vi "Next Message.vi"(7 "Periodic Name (None = Timeout)":string, 8 "error in (no error)":errorcluster, 9 "Timeout/Period ms (-1)":i32=-1, 11 "Module in":refnum<class "Module.lvclass">) -> (0 "error out":errorcluster, 1 "Data":variant, 2 "ID":string, 3 "Module out":refnum<class "Module.lvclass">)   [LabVIEW 2023, in "Volatus.lvlib" / "Module.lvclass"]
uses:
  Module.lvclass
  Module.lvclass/Module.ctl
  MessageQ/MessageQ.lvclass/MessageQ.ctl
  Module Status Update.ctl
  MessageQ/MessageQ.lvclass
  State.ctl
  Module Substatus.ctl
  Metric Update.ctl
  Launch Nested Message.ctl
  VolatusConfig/VolatusConfigElement/VolatusConfigElement.lvclass
  LastAck.ctl
  MessageQ/Send.vi
  Parent Q.vi
  MessageQ/Is Null.vi
  Volatus.lvlib
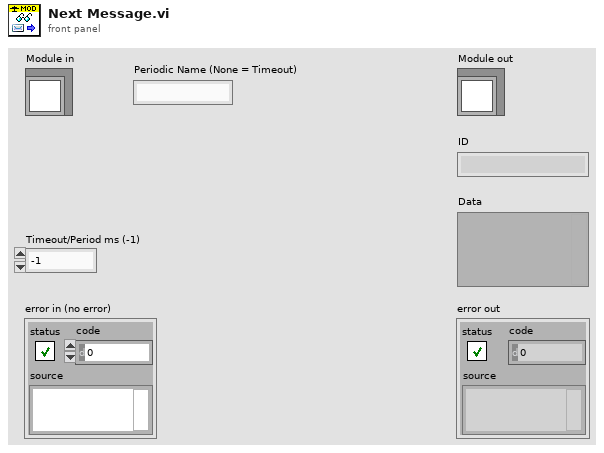
[diagram p1: front panel]
types:
  T1 = typedef "Volatus.lvlib/Metrics Reverse.ctl" = cluster{"End HRS":dbl, "Wait":dbl}
  T2 = typedef "Volatus.lvlib/Metrics Forward.ctl" = cluster{"Name":string, "Start":dbl, "Proc":dbl}
  T3 = typedef "Volatus.lvlib/Module Status Update.ctl" = cluster{"MessageQ":refnum<class "MessageQ.lvclass">, "State":T4, "Hierarchy":string[], "Forwarded":bool}
  T4 = typedef "Volatus.lvlib/Module.lvclass/State.ctl" = enum16{"Unknown", "Launched", "Starting", "Running", "Stopping", "Stopped", "Error - Starting", "Error - Run", "Error - Stopping"}
  T5 = typedef "Volatus.lvlib/Module Substatus.ctl" = cluster{"Hierarchy":string[], "Name":string, "Status":string}
  T6 = typedef "Volatus.lvlib/Metric Update.ctl" = cluster{"Hierarchy":string[], "Name":string, "Value":dbl}
  T7 = typedef "Volatus.lvlib/Launch Nested Message.ctl" = cluster{"Module":refnum<class "Module.lvclass">, "Config":refnum<class "VolatusConfigElement.lvclass">}
  T8 = typedef "Volatus.lvlib/Module.lvclass/LastAck.ctl" = cluster{"Module":refnum<class "Module.lvclass">}
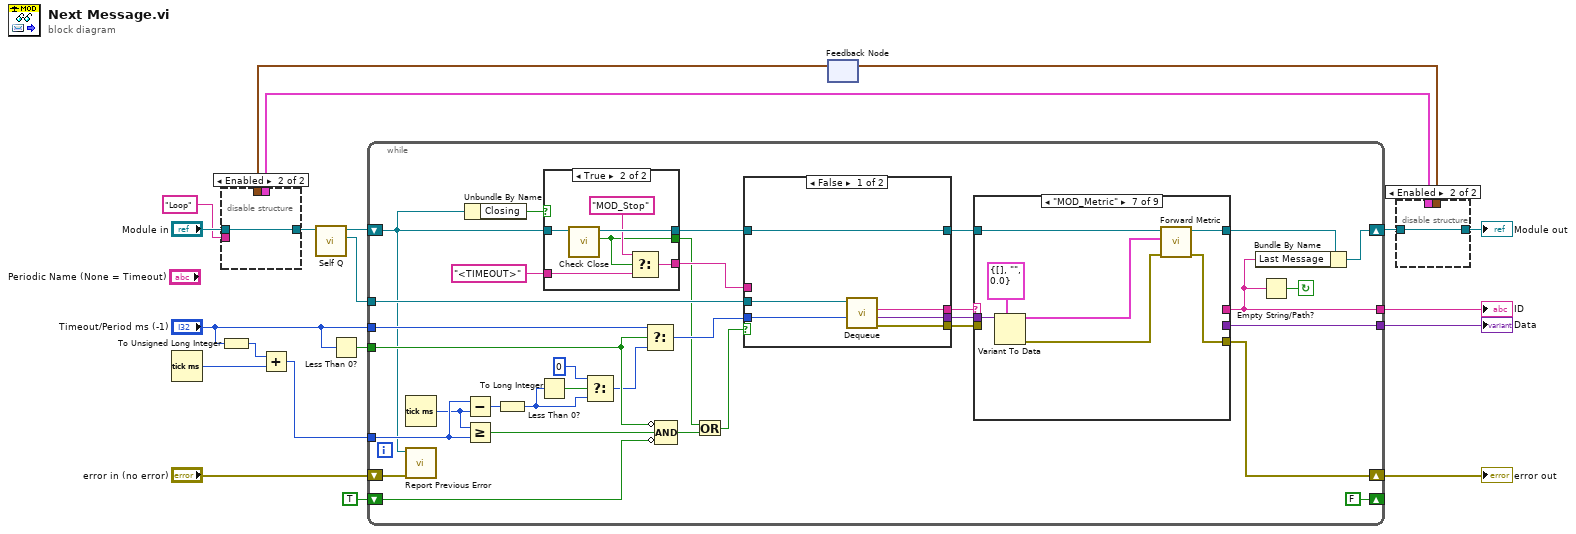
[diagram p0: block diagram]
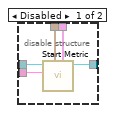
[diagram p2: hidden frame]
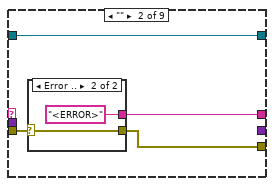
[diagram p6: hidden frame]
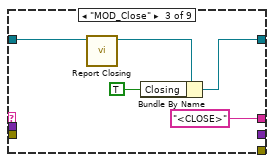
[diagram p8: hidden frame]
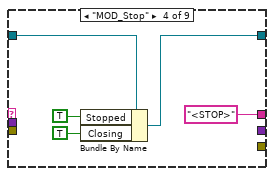
[diagram p9: hidden frame]
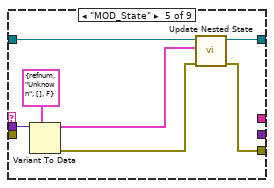
[diagram p10: hidden frame]
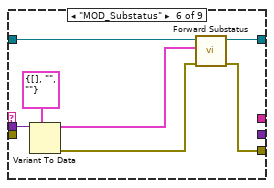
[diagram p11: hidden frame]
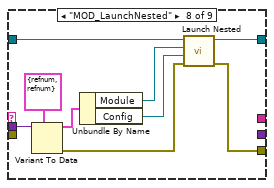
[diagram p12: hidden frame]
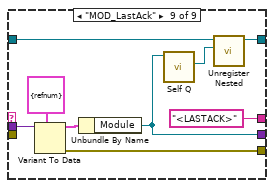
[diagram p13: hidden frame]
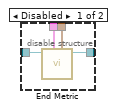
[diagram p14: hidden frame]
diagram:
  n1 = Tick Count (ms)() -> (millisecond timer value=w3:u32)
  n2 = To Unsigned Long Integer(number="Timeout/Period ms (-1)") -> (unsigned 32bit integer=w2:u32)
  n3 = Add(x=w2, y=w3) -> (x+y=w1:u32)
  n4 = Less Than 0?(x="Timeout/Period ms (-1)") -> (x < 0?=w6:bool)
  n5 = feedback #1() -> (w9:T1)  [unwired: 1 in]
  n6 = disable-structure shown="Enabled" {
    disable-tunnel: "Module in" -> [w25 w26]
    disable-tunnel: [w24 w26] -> w14
    disable-tunnel: "Loop" ("Metric") -> [w23 _]
    disable-tunnel: [w22 _] -> w11
    disable-tunnel: w9 -> [w21 _]
    frame Disabled {
      n7 = call "Start Metric.vi"("Metrics Reverse"=w21, "Metric"=w23, "Module in"=w25) -> ("Module out"=w24:refnum<class "Module.lvclass">, "Forward"=w22:T2)  [unwired: 6 in, 1 out]
    }
    frame Enabled {
    }
  }
  n8 = call "Self Q.vi"("Module in"=w14) -> ("Self Q"=w7:refnum<class "MessageQ.lvclass">, "Module out"=w8:refnum<class "Module.lvclass">)  [unwired: 9 in]
  n9 = while {
    shift-right: [w43] -> w15
    shift-left: w8 -> [w32]
    tunnel: w7 -> [w58]
    tunnel: w1 -> [w49]
    tunnel: [w45] -> w16
    tunnel: [w53] -> w19
    tunnel: "Timeout/Period ms (-1)" -> [w51]
    tunnel: w6 -> [w41]
    shift-right: [w46] -> w17
    shift-left: "error in (no error)" -> [w59]
    shift-right: [FALSE] -> _
    shift-left: TRUE -> [w39]
    stop <- w52 continue-if-true
    n10 = Tick Count (ms)() -> (millisecond timer value=w48:u32)
    n11 = call "Report Previous Error.vi"("error in (no error)"=w59, "Module in"=w32) -> ()  [unwired: 8 in, 2 out]
    n12 = Unbundle By Name(w32) -> ("Closing"=w34:bool)
    n13 = Subtract(x=w49, y=w48) -> (x-y=w57:u32)
    n14 = Greater Or Equal?(x=w48, y=w49) -> (x >= y?=w47:bool)
    n15 = To Long Integer(number=w57) -> (32bit integer=w36:i32)
    n16 = Less Than 0?(x=w36) -> (x < 0?=w38:bool)
    n17 = case shown="True" w34 {
      tunnel: w32 -> [w61 w67]
      tunnel: [w61 w66] -> w29
      tunnel: "<TIMEOUT>" ("ID") -> [w60 w65]
      tunnel: [w60 w63] -> w33
      tunnel: [_ w62] -> w30
      frame False {
      }
      frame True {
        n18 = call "Check Close.vi"("Module in"=w67) -> ("Stop"=w62:bool, "Module out"=w66:refnum<class "Module.lvclass">)  [unwired: 8 in, 1 out]
        n19 = Select(t="MOD_Stop", s=w62, f=w65) -> (s? t:f=w63:string)
      }
    }
    n20 = Select(t=0 ("32bit integer"), s=w38, f=w36) -> (s? t:f=w35:i32)
    n21 = Select(t=w51, s=w41, f=w35) -> (s? t:f=w50:i32)
    n22 = Compound Arithmetic op=AND(invert w41, w47, invert w39) -> (w42:bool)
    n23 = Or(x=w30, y=w42) -> (x .or. y?=w31:bool)
    n24 = case shown="False" w31 {
      tunnel: w58 -> [w72 _]
      tunnel: [w71 w75] -> w56
      tunnel: [w70 _] -> w55
      tunnel: [w73 _] -> w54
      tunnel: w50 -> [w69 _]
      tunnel: w33 -> [_ w75]
      tunnel: w29 -> [w68 w74]
      tunnel: [w68 w74] -> w28
      frame False {
        n25 = call "Dequeue.vi"("Timeout ms (-1)"=w69, "MessageQ in"=w72) -> ("error out"=w73:errorcluster, "Data"=w70:variant, "ID"=w71:string)  [unwired: 6 in, 1 out]
      }
      frame True {
      }
    }
    n26 = case shown="\"MOD_Metric\"" w56 {
      selector: w56 -> [w78 _ _ _ _ _ _ _ _]
      tunnel: w55 -> [w76 _ _ _ w101 w108 w115 w124 w133]
      tunnel: w54 -> [_ w80 _ _ _ _ _ _ _]
      tunnel: w28 -> [w77 w82 w89 w93 w99 w106 w113 w121 w127]
      tunnel: [w77 w82 w87 w92 w98 w105 w112 w120 w129] -> w44
      tunnel: [w78 w81 "<CLOSE>" "<STOP>" _ _ _ _ "<LASTACK>"] -> w45
      tunnel: [w76 _ _ _ _ _ _ _ w126] -> w53
      tunnel: [_ w79 _ _ w97 w104 w111 w116 w125] -> w46
      frame Default {
      }
      frame "" {
        n27 = case shown="Error .." w80 {
          selector: w80 -> [_ w83]
          tunnel: [_ "<ERROR>"] -> w81
          tunnel: [_ w83] -> w79
          frame No Error {
          }
          frame Error {
          }
        }
      }
      frame "MOD_Close" {
        n28 = call "Report Closing.vi"("Module in"=w89) -> ("Module out"=w85:refnum<class "Module.lvclass">)  [unwired: 9 in, 1 out]
        n29 = Bundle By Name(cluster=w85, "Closing"=TRUE) -> (w87:refnum<class "Module.lvclass">)
      }
      frame "MOD_Stop" {
        n30 = Bundle By Name(cluster=w93, "Stopped"=TRUE, "Closing"=TRUE) -> (w92:refnum<class "Module.lvclass">)
      }
      frame "MOD_State" {
        n31 = Variant To Data(type=T3 {"MessageQ"=refnum, "State"=enum."Unknown", "Hierarchy"=[], "Forwarded"=FALSE} ("Nested State Data"), Variant=w101) -> (data=w95:T3, error out=w96:errorcluster)  [unwired: 1 in]
        n32 = call "Update Nested State.vi"("error in (no error)"=w96, "Module Status"=w95, "Module in"=w99) -> ("error out"=w97:errorcluster, "Module out"=w98:refnum<class "Module.lvclass">)  [unwired: 7 in]
      }
      frame "MOD_Substatus" {
        n33 = Variant To Data(type=T5 {"Hierarchy"=[], "Name"="", "Status"=""} ("Nested State Data"), Variant=w108) -> (data=w102:T5, error out=w103:errorcluster)  [unwired: 1 in]
        n34 = call "Forward Substatus.vi"("error in (no error)"=w103, "Module Substatus"=w102, "Module in"=w106) -> ("error out"=w104:errorcluster, "Module out"=w105:refnum<class "Module.lvclass">)  [unwired: 7 in]
      }
      frame "MOD_Metric" {
        n35 = Variant To Data(type=T6 {"Hierarchy"=[], "Name"="", "Value"=0.0} ("Nested State Data"), Variant=w115) -> (data=w109:T6, error out=w110:errorcluster)  [unwired: 1 in]
        n36 = call "Forward Metric.vi"("error in (no error)"=w110, "Metric Update"=w109, "Module in"=w113) -> ("error out"=w111:errorcluster, "Module out"=w112:refnum<class "Module.lvclass">)  [unwired: 7 in]
      }
      frame "MOD_LaunchNested" {
        n37 = Variant To Data(type=T7 {"Module"=refnum, "Config"=refnum} ("Launch Nested Message"), Variant=w124) -> (data=w122:T7, error out=w117:errorcluster)  [unwired: 1 in]
        n38 = Unbundle By Name(w122) -> ("Module"=w119:refnum<class "Module.lvclass">, "Config"=w118:refnum<class "VolatusConfigElement.lvclass">)
        n39 = call "Launch Nested.vi"("error in (no error)"=w117, "Config Element"=w118, "Nested Module"=w119, "Parent in"=w121) -> ("error out"=w116:errorcluster, "Parent out"=w120:refnum<class "Module.lvclass">)  [unwired: 5 in, 1 out]
      }
      frame "MOD_LastAck" {
        n40 = Variant To Data(type=T8 {"Module"=refnum} ("LastAck"), Variant=w133) -> (data=w131:T8, error out=w125:errorcluster)  [unwired: 1 in]
        n41 = Unbundle By Name(w131) -> ("Module"=w126:refnum<class "Module.lvclass">)
        n42 = call "Self Q.vi"("Module in"=w126) -> ("Self Q"=w130:refnum<class "MessageQ.lvclass">)  [unwired: 9 in, 1 out]
        n43 = call "Unregister Nested.vi"("MessageQ"=w130, "Module in"=w127) -> ("Module out"=w129:refnum<class "Module.lvclass">)  [unwired: 8 in, 1 out]
      }
    }
    n44 = Bundle By Name(cluster=w44, "Last Message"=w45) -> (w43:refnum<class "Module.lvclass">)
    n45 = Empty String/Path?(string/path=w45) -> (empty?=w52:bool)
  }
  "error out" <- w17
  "ID" <- w16
  "Data" <- w19
  n46 = disable-structure shown="Enabled" {
    disable-tunnel: w15 -> [w137 w138]
    disable-tunnel: [w136 w138] -> w13
    disable-tunnel: w11 -> [w135 _]
    disable-tunnel: [w134 _] -> w10
    frame Disabled {
      n47 = call "End Metric.vi"("Metrics Forward"=w135, "Module in"=w137) -> ("Module out"=w136:refnum<class "Module.lvclass">, "Metrics Reverse"=w134:T1)  [unwired: 7 in, 1 out]
    }
    frame Enabled {
    }
  }
  "Module out" <- w13
  n48 = feedback-in #1(w10) -> ()
